vi "MultiChannelfFeedbackCooling (FPGA).vi"() -> ()   [LabVIEW 2016]
doc: "This VI will read single point values from 4 channels of a R Series board at a specified rate."
uses:
  <vilib>/rvi/Emulation/niFpgaGetClockAttributes.vi
  <vilib>/rvi/Emulation/niFpgaSctlEmulationGetInTimedLoop.vi
  <vilib>/rvi/Emulation/niFpgaEmulationReportErrorSimple.vi
  <vilib>/rvi/eio/common/nirviEmuTemplateMethod_errors.vi
  <vilib>/rvi/Memory/Memory_Emulation/nirvimemoryFastEmulation.vi
  <vilib>/rvi/Memory/Memory_Emulation/nirvimemoryEmulation.vi
  <vilib>/rvi/Emulation/niFpgaEmulationIsFPGAContextNoSignature.vi
  <vilib>/rvi/DataTransferAndStorage/Container/Common/niFpgaContainerGetUniqueNameForEmu.vi
  <vilib>/rvi/Emulation/niFpgaProcessEmulError.vi
  <vilib>/rvi/errors/nirviReportUnexpectedCaseInternalError (U32).vi
  <vilib>/rvi/Memory/Memory_Emulation/niFpgaMemoryEmulationCacheClearOnFirstRun.vi
  <vilib>/rvi/Memory/Memory_Emulation/nirvimemoryEmulationManagerCache_MakeExclusive.vi
  <vilib>/rvi/Memory/Memory_Emulation/niFpgaMemoryEmulationValidateCache.vi
  <vilib>/rvi/Memory/Memory_Emulation/nirvimemoryEmulationManagerCache_InsertValue.vi
  <vilib>/Utility/error.llb/Clear Errors.vi
  <vilib>/rvi/Memory/Memory_Emulation/nirvimemoryEmulationManagerCache_ReleaseExclusive.vi
  <vilib>/rvi/Memory/Memory_Emulation/nirvimemoryEmulationManagerCache_GetValue.vi
  <vilib>/rvi/Memory/Memory_Emulation/nirvimemoryEmulationManagerCache_SetValue.vi
  <vilib>/rvi/Emulation/niFpgaSctlEmulationResourceMgr.vi
  <vilib>/rvi/Emulation/niFpgaCriticalErrorInLSC.vi
  <vilib>/eio/EIONode/EIONode.xnode
  <vilib>/rvi/DataTransferAndStorage/Container/XNode/niFpgaContainer.xnode
  <vilib>/rvi/FXPMathLib/FxpInterpret/XNode/nifxpmath_Interpret.xnode
panel:
  in  "pg d0 1":fxp<+/-,24,12>
  in  "dg d0 1":fxp<+/-,24,12>
  in  "ig d0 1":fxp<+/-,24,6>
  in  "Upper lim d0 1":fxp<+/-,16,16>
  in  "Lower lim 2a":fxp<+/-,16,16>
  out "AI3":i16
  in  "lp coeff d0":i32[](array[numeric])=[1008310688, 32715568]
  in  "hp coeff d0":i32[](array[numeric])=[946630756, 1010186290]
  in  "Dc Pos d0":i16
  out "fb_d0":i16
  in  "Use_PID0_X":bool
  out "AI4":i16
  in  "Use_PID1_X":bool
  in  "Dc Pos d1":i16
  out "fb_d1":i16
  in  "Lower lim 3":fxp<+/-,16,16>
  in  "Upper lim d0 2":fxp<+/-,16,16>
  in  "pg d0 2":fxp<+/-,24,12>
  in  "hp coeff d1":i32[](array[numeric])=[946630756, 1010186290]
  in  "dg d0 2":fxp<+/-,24,12>
  in  "ig d0 2":fxp<+/-,24,6>
  in  "lp coeff d1":i32[](array[numeric])=[1008310688, 32715568]
  in  "ig 0":fxp<+/-,24,6>
  in  "pg 0":fxp<+/-,24,12>
  in  "ig 1":fxp<+/-,24,6>
  in  "pg 1":fxp<+/-,24,12>
  in  "pg_img":fxp<+/-,24,12>
  in  "dg_img":fxp<+/-,24,12>
  in  "ig_img":fxp<+/-,24,6>
  in  "setpt_img":i16
  out "AI_img":i16
  in  "lp coeff_img":i32[](array[numeric])=[1008310688, 32715568]
  in  "Upper lim_img":fxp<+/-,16,16>
  in  "Lower lim_img":fxp<+/-,16,16>
  in  "lp coeff d2":i32[](array[numeric])=[1008310688, 32715568]
  in  "hp coeff_img":i32[](array[numeric])=[946630756, 1010186290]
  out "tot_fb_img":i16
  out "fb_img":i16
  in  "output offset_img":i16
  in  "lp coeff 2":i32[](array[numeric])=[1008310688, 32715568]
  in  "data_buffer3":i16
  in  "Arb gain (ch2)":fxp<+/-,24,12>=0.5 caption="RMS"
  in  "lp coeff 0":i32[](array[numeric])=[1008310688, 32715568]
  in  "lp coeff 1":i32[](array[numeric])=[1008310688, 32715568]
  in  "hp coeff d2":i32[](array[numeric])=[946630756, 1010186290]
  in  "hp coeff 2":i32[](array[numeric])=[946630756, 1010186290]
  in  "hp coeff 1":i32[](array[numeric])=[946630756, 1010186290]
  in  "hp coeff 0":i32[](array[numeric])=[946630756, 1010186290]
  in  "Use_PID2_X 2":bool
  out "AI5":i16
  in  "Dc Pos d2":i16
  out "tot_fb_2":i16
  out "tot_fb_1":i16
  out "tot_fb_0":i16
  out "fb_d2":i16
  in  "output offset 2":i16
  in  "output offset 1":i16
  in  "output offset 0":i16
  in  "Lower lim 4":fxp<+/-,16,16>
  in  "Upper lim d0 3":fxp<+/-,16,16>
  in  "pg d0 3":fxp<+/-,24,12>
  in  "ig d03":fxp<+/-,24,6>
  in  "dg d0 3":fxp<+/-,24,12>
  out "fb_2":i16
  in  "ig 3":fxp<+/-,24,6>
  out "written_address":u32
  in  "ready_to_write":bool
  in  "Arb steps per cycle":u16
  in  "data_buffer2":i16
  in  "data_buffer_1":i16
  in  "write_address":u16
  in  "Arb gain (ch1)":fxp<+/-,24,12>=0.5 caption="RMS"
  in  "Arb gain (ch0)":fxp<+/-,24,12>=0.5 caption="RMS"
  out "fb_1":i16
  out "fb_0":i16
  in  "Dc Pos 1":i16
  in  "Dc Pos 0":i16
  in  "Lower lim 2":fxp<+/-,16,16>
  in  "Upper lim 2":fxp<+/-,16,16>
  in  "dg 2":fxp<+/-,24,12>
  in  "pg 2":fxp<+/-,24,12>
  out "AI2":i16
  in  "Dc Pos 2":i16
  out "AI1":i16
  in  "dg 1":fxp<+/-,24,12>
  in  "Upper lim 1":fxp<+/-,16,16>
  in  "Lower lim 1":fxp<+/-,16,16>
  out "AI0":i16
  in  "dg 0":fxp<+/-,24,12>
  in  "Upper lim 0":fxp<+/-,16,16>
  in  "Lower lim 0":fxp<+/-,16,16>
  in  "Count(uSec)":u32
  out "FPGA Error Out":errorcluster
  in  "Stop":bool
  # "test"
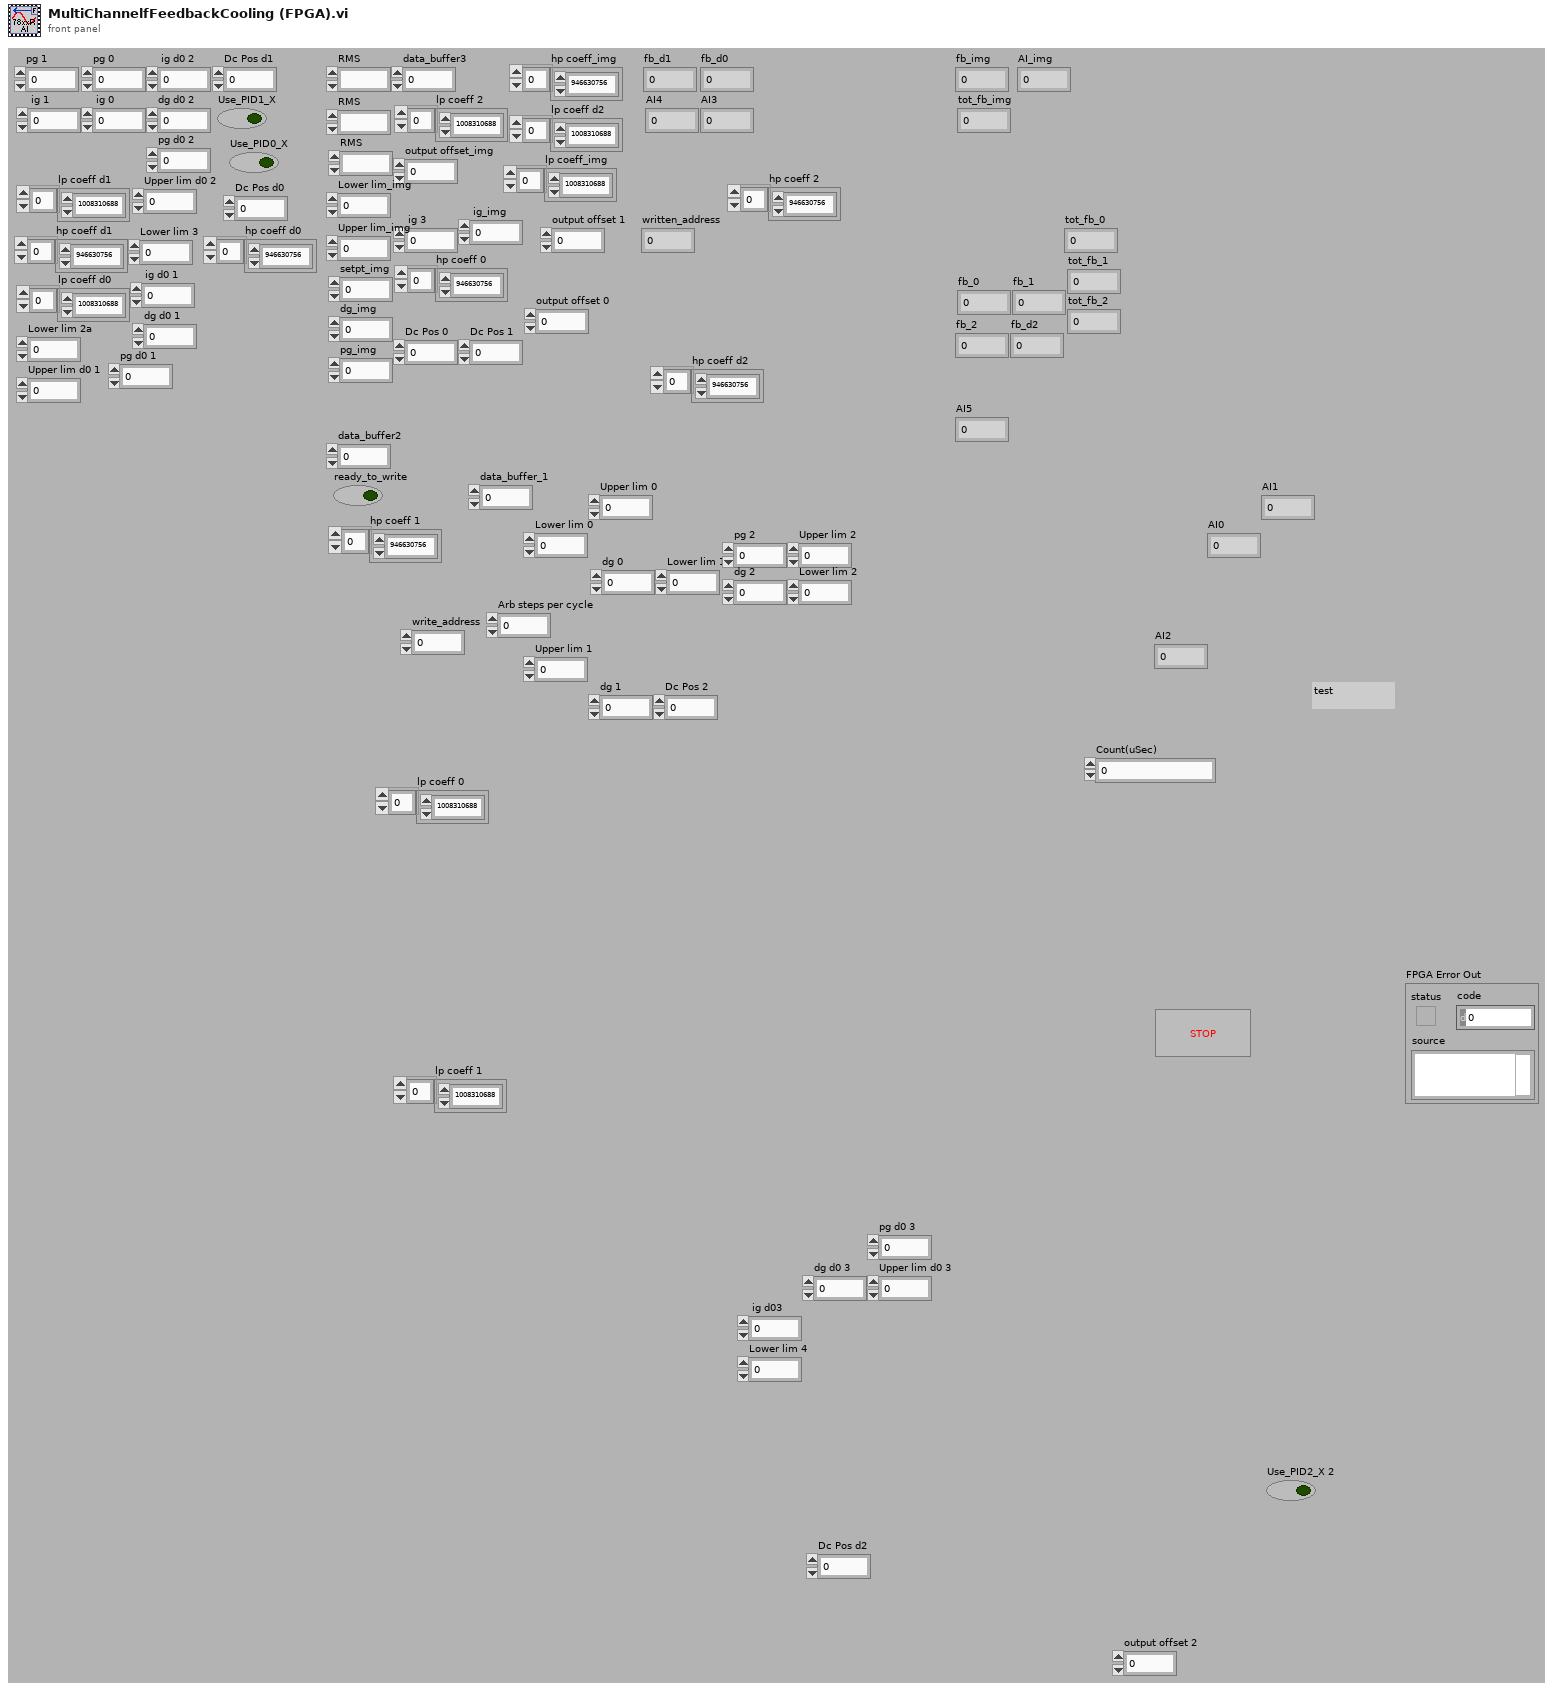
[diagram p1: front panel]
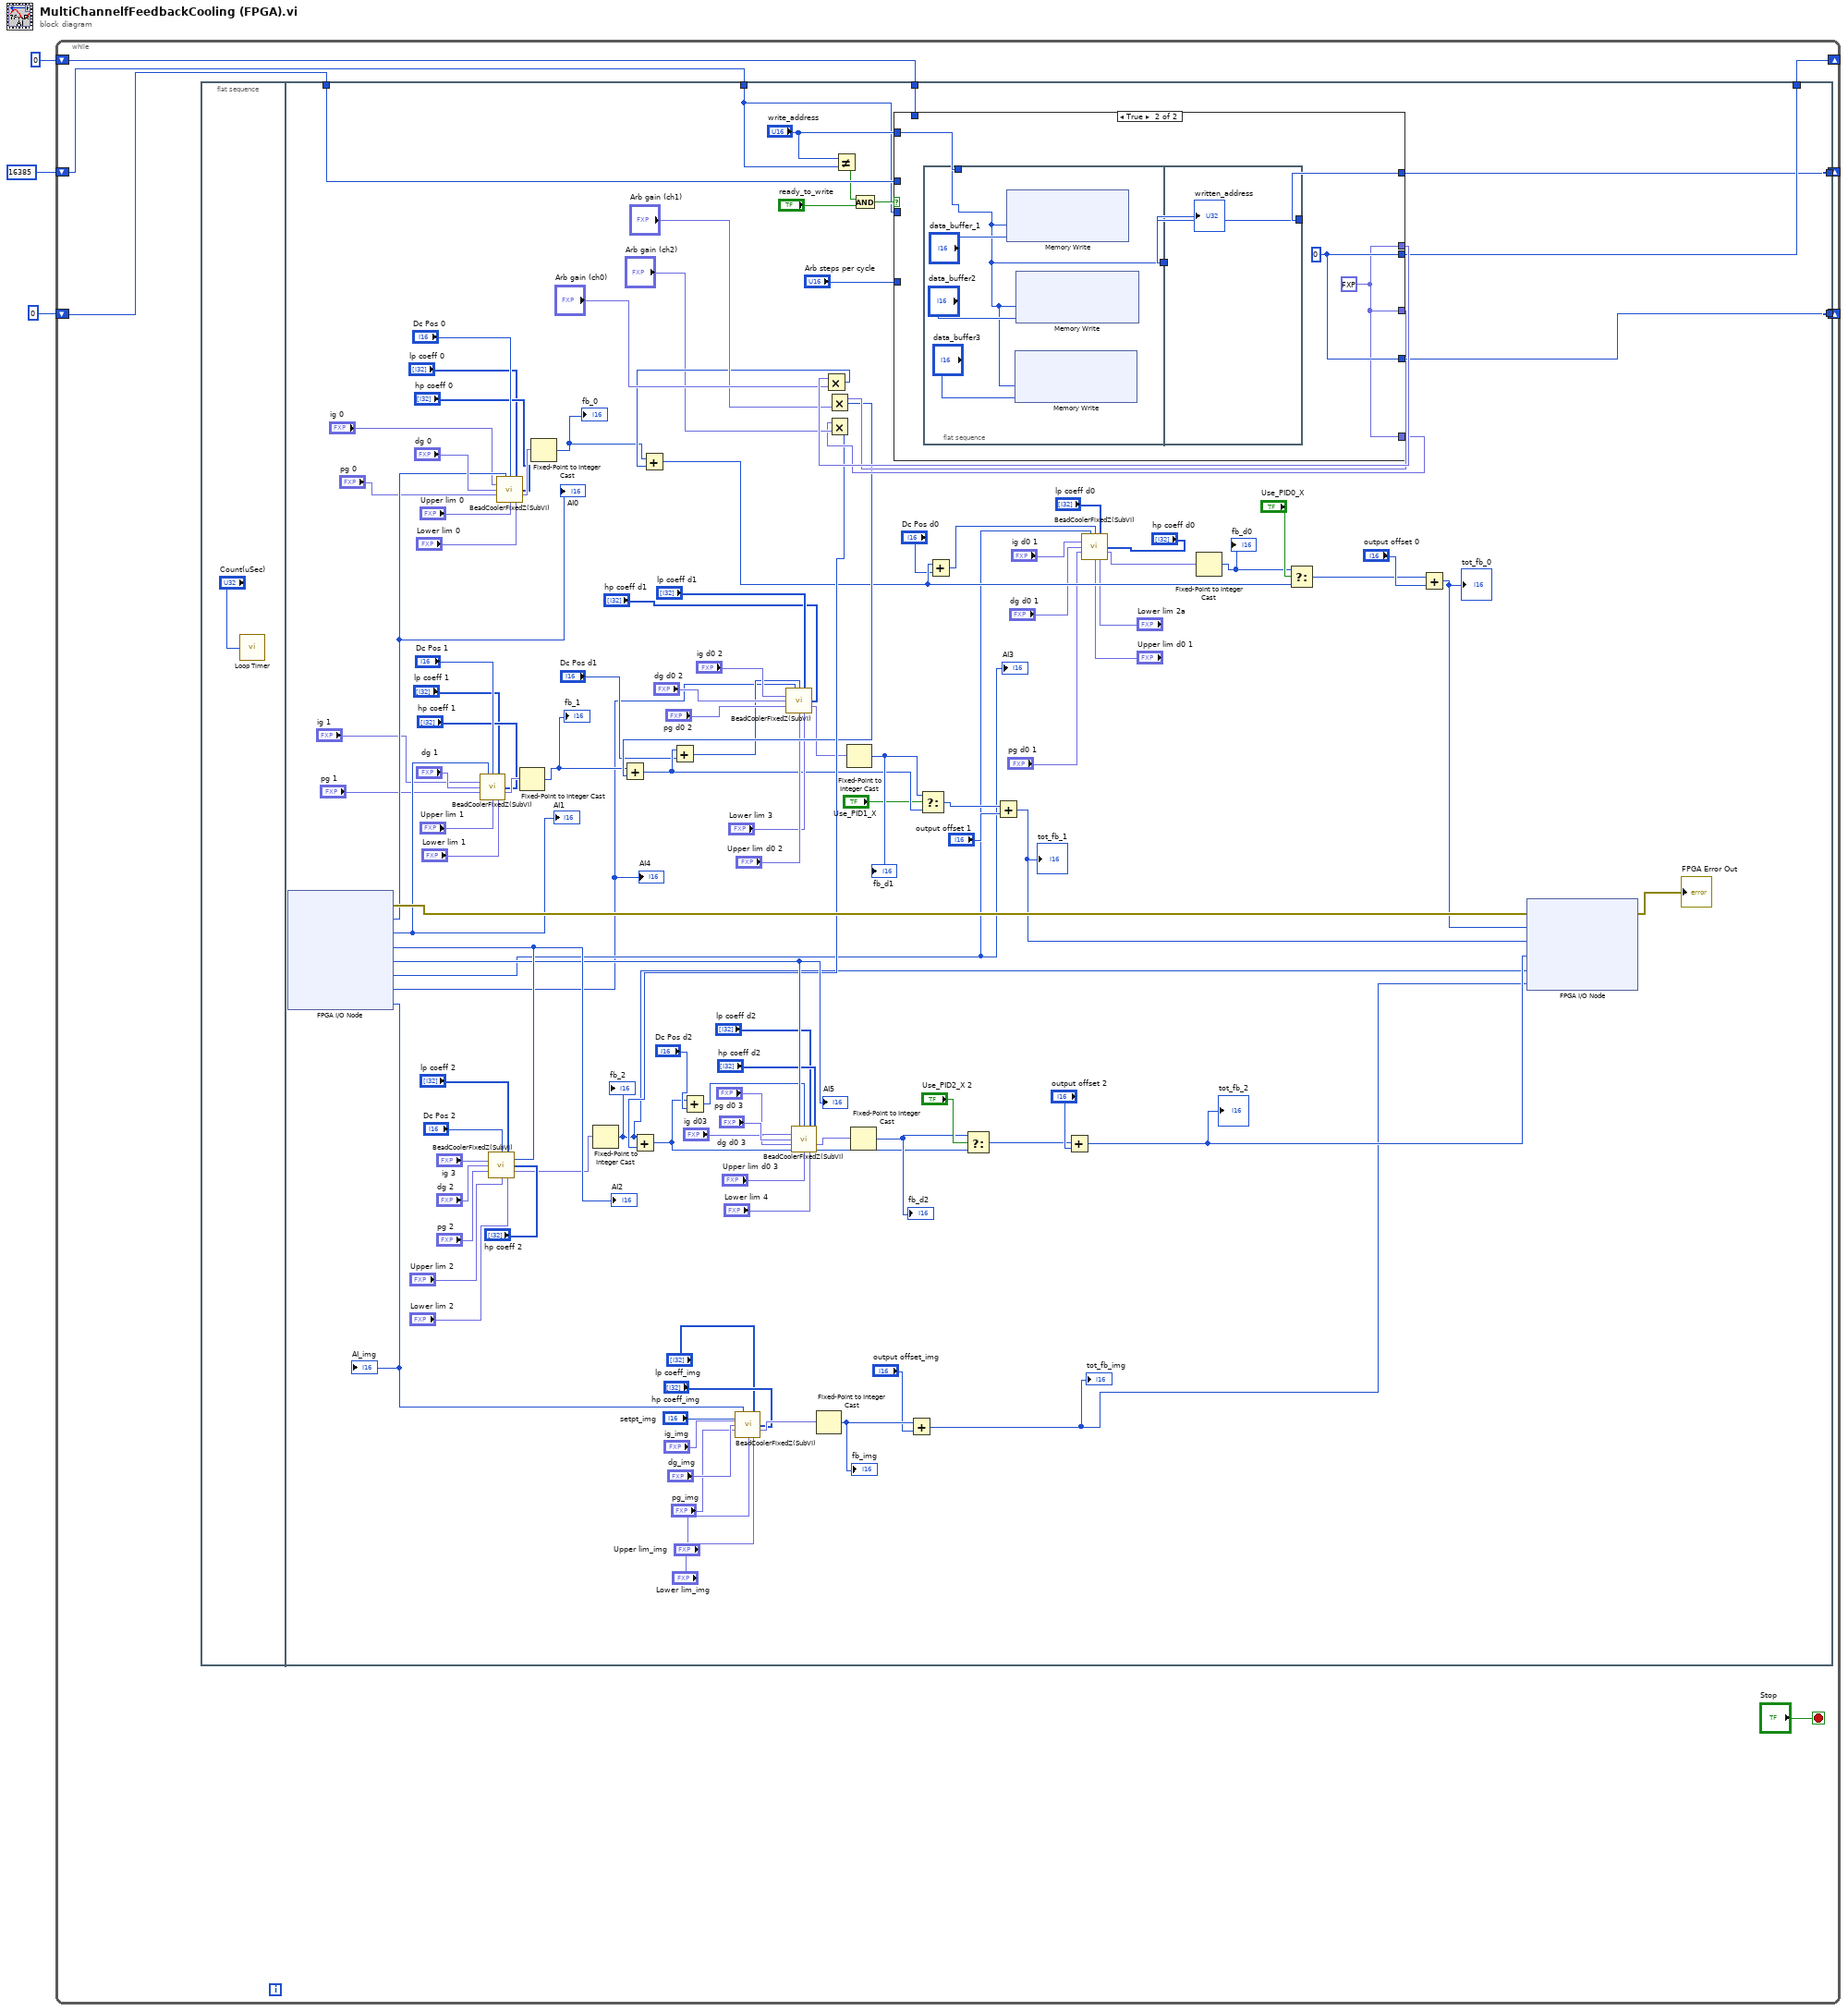
[diagram p0: block diagram]
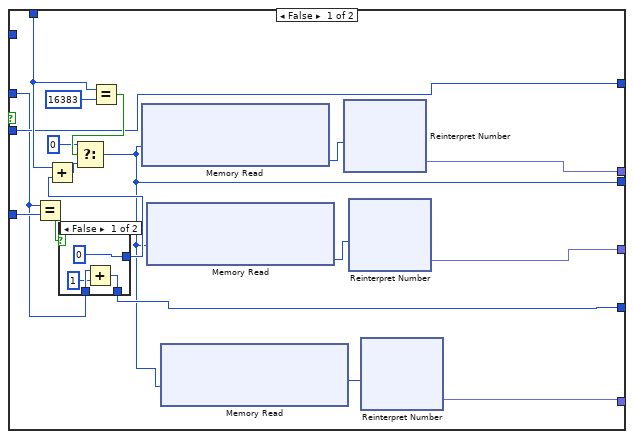
[diagram p2: hidden frame]
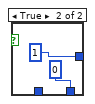
[diagram p3: hidden frame]
diagram:
  n1 = while {
    shift-right: [w9] -> _
    shift-left: u16 0 ("t") -> [w8]
    shift-right: [w7] -> _
    shift-left: u16 0 ("t") -> [w4]
    shift-right: [w6] -> _
    shift-left: u32 16385 ("write_address") -> [w5]
    stop <- "Stop" stop-if-true
    n2 = flat-sequence {
      tunnel: [w113] -> w9
      tunnel: w8 -> [w112]
      tunnel: [w110] -> w7
      tunnel: w4 -> [w109]
      tunnel: [w108] -> w6
      tunnel: w5 -> [w100]
      frame #0 {
        n3 = call "Loop Timer"("Count(uSec)"="Count(uSec)") -> ()  [unwired: 1 out]
      }
      frame #1 {
        n4 = xnode "FPGA I/O Node"() -> ("error out"=w130:errorcluster, "Connector0/AI0"=w99:i16, "Connector0/AI1"=w98:i16, "Connector0/AI2"=w95:i16, "Connector0/AI5"=w83:i16, "Connector0/AI3"=w18:i16, "Connector0/AI4"=w12:i16, "Connector0/AI6"=w49:i16)  [unwired: 8 in, 7 out]
        "AI0" <- w99
        "AI1" <- w98
        "AI2" <- w95
        "AI5" <- w83
        "AI_img" <- w49
        "AI4" <- w12
        "AI3" <- w18
        n5 = call "BeadCoolerFixedZ(SubVI).vi"("AI0"=w98, "Dc Pos"="Dc Pos 1", "lp coeff"="lp coeff 1", "ig"="ig 1", "dg"="dg 1", "hp coeff"="hp coeff 1", "pg"="pg 1", "Upper lim"="Upper lim 1", "Lower lim"="Lower lim 1") -> ("Output"=w97:fxp<+/-,16,16>)  [unwired: 6 in]
        n6 = call "BeadCoolerFixedZ(SubVI).vi"("AI0"=w95, "Dc Pos"="Dc Pos 2", "lp coeff"="lp coeff 2", "ig"="ig 3", "dg"="dg 2", "hp coeff"="hp coeff 2", "pg"="pg 2", "Upper lim"="Upper lim 2", "Lower lim"="Lower lim 2") -> ("Output"=w73:fxp<+/-,16,16>)  [unwired: 6 in]
        n7 = call "BeadCoolerFixedZ(SubVI).vi"("AI0"=w99, "Dc Pos"="Dc Pos 0", "lp coeff"="lp coeff 0", "ig"="ig 0", "dg"="dg 0", "hp coeff"="hp coeff 0", "pg"="pg 0", "Upper lim"="Upper lim 0", "Lower lim"="Lower lim 0") -> ("Output"=w101:fxp<+/-,16,16>)  [unwired: 6 in]
        n8 = Fixed-Point to Integer Cast(1:w97) -> (0:w30:i16)
        "fb_1" <- w30
        n9 = Fixed-Point to Integer Cast(1:w101) -> (0:w68:i16)
        "fb_0" <- w68
        n10 = Fixed-Point to Integer Cast(1:w73) -> (0:w36:i16)
        "fb_2" <- w36
        n11 = call "BeadCoolerFixedZ(SubVI).vi"("AI0"=w49, "Dc Pos"="setpt_img", "lp coeff"="lp coeff_img", "ig"="ig_img", "dg"="dg_img", "hp coeff"="hp coeff_img", "pg"="pg_img", "Upper lim"="Upper lim_img", "Lower lim"="Lower lim_img") -> ("Output"=w62:fxp<+/-,16,16>)  [unwired: 6 in]
        n12 = Fixed-Point to Integer Cast(1:w62) -> (0:w61:i16)
        "fb_img" <- w61
        n13 = Not Equal?(x="write_address", y=w100) -> (x != y?=w105:bool)
        n14 = And(x=w105, y="ready_to_write") -> (x .and. y?=w106:bool)
        n15 = case shown="True" w106 {
          tunnel: [w147 w155] -> w115
          tunnel: [w132 w159] -> w113
          tunnel: w112 -> [w140 _]
          tunnel: [w141 w155] -> w103
          tunnel: "Arb steps per cycle" -> [w139 _]
          tunnel: [w134 w159] -> w110
          tunnel: w109 -> [w135 _]
          tunnel: [w138 w157] -> w108
          tunnel: w100 -> [w138 _]
          tunnel: "write_address" -> [_ w156]
          tunnel: [w131 w155] -> w66
          frame False {
            n16 = Equal?(x=w135, y=w139) -> (x = y?=w137:bool)
            n17 = case shown="False" w137 {
              tunnel: [u16 0 ("y") u16 1 ("y")] -> w136
              tunnel: w135 -> [w151 _]
              tunnel: [w149 u16 0] -> w134
              frame False {
                n18 = Add(x=w151, y=u16 1) -> (x+y=w149:u16)
              }
              frame True {
              }
            }
            n19 = Add(x=w140, y=w136) -> (x+y=w143:u16)
            n20 = Equal?(x=w140, y=u16 16383) -> (x = y?=w145:bool)
            n21 = Select(t=u16 0, s=w145, f=w143) -> (s? t:f=w132:u16)
            n22 = xnode ("Memory Read")("Address"=w132) -> ("Data"=w148:i16)  [unwired: 1 in, 1 out]
            n23 = xnode ("Memory Read")("Address"=w132) -> ("Data"=w142:i16)  [unwired: 1 in, 1 out]
            n24 = xnode ("Memory Read")("Address"=w132) -> ("Data"=w133:i16)  [unwired: 1 in, 1 out]
            n25 = xnode "Reinterpret Number"("x"=w148) -> ("y"=w147:fxp<+/-,16,16>)
            n26 = xnode "Reinterpret Number"("x"=w142) -> ("y"=w141:fxp<+/-,16,16>)
            n27 = xnode "Reinterpret Number"("x"=w133) -> ("y"=w131:fxp<+/-,16,16>)
          }
          frame True {
            w159 = u16 0
            w155 = fxp<+/-,16,16> 0.0 ("y")
            n28 = flat-sequence {
              tunnel: [w161] -> w158
              tunnel: w156 -> [w161]
              tunnel: w158 -> [w164]
              tunnel: [w164] -> w157
              frame #0 {
                n29 = xnode ("Memory Write")("Address"=w161, "Data"="data_buffer_1") -> ()  [unwired: 1 in, 1 out]
                n30 = xnode ("Memory Write")("Address"=w161, "Data"="data_buffer3") -> ()  [unwired: 1 in, 1 out]
                n31 = xnode ("Memory Write")("Address"=w161, "Data"="data_buffer2") -> ()  [unwired: 1 in, 1 out]
              }
              frame #1 {
                "written_address" <- w164
              }
            }
          }
        }
        n32 = Multiply(x=w115, y="Arb gain (ch0)") -> (x*y=w87:i16)
        n33 = Add(x=w68, y=w87) -> (x+y=w22:i16)
        n34 = Multiply(x=w103, y="Arb gain (ch1)") -> (x*y=w64:i16)
        n35 = Add(x=w30, y=w64) -> (x+y=w33:i16)
        n36 = Add(x=w33, y="Dc Pos d1") -> (x+y=w31:i16)
        n37 = call "BeadCoolerFixedZ(SubVI).vi"("AI0"=w12, "Dc Pos"=w31, "lp coeff"="lp coeff d1", "ig"="ig d0 2", "dg"="dg d0 2", "hp coeff"="hp coeff d1", "pg"="pg d0 2", "Upper lim"="Upper lim d0 2", "Lower lim"="Lower lim 3") -> ("Output"=w37:fxp<+/-,16,16>)  [unwired: 6 in]
        n38 = Multiply(x=w66, y="Arb gain (ch2)") -> (x*y=w65:i16)
        n39 = Add(x=w36, y=w65) -> (x+y=w72:i16)
        n40 = Add(x=w72, y="Dc Pos d2") -> (x+y=w69:i16)
        n41 = call "BeadCoolerFixedZ(SubVI).vi"("AI0"=w83, "Dc Pos"=w69, "lp coeff"="lp coeff d2", "ig"="ig d03", "dg"="dg d0 3", "hp coeff"="hp coeff d2", "pg"="pg d0 3", "Upper lim"="Upper lim d0 3", "Lower lim"="Lower lim 4") -> ("Output"=w89:fxp<+/-,16,16>)  [unwired: 6 in]
        n42 = Fixed-Point to Integer Cast(1:w37) -> (0:w34:i16)
        "fb_d1" <- w34
        n43 = Fixed-Point to Integer Cast(1:w89) -> (0:w80:i16)
        "fb_d2" <- w80
        n44 = Add(x=w61, y="output offset_img") -> (x+y=w60:i16)
        "tot_fb_img" <- w60
        n45 = Select(t=w34, s="Use_PID1_X", f=w33) -> (s? t:f=w35:i16)
        n46 = Add(x=w22, y="Dc Pos d0") -> (x+y=w23:i16)
        n47 = Select(t=w80, s="Use_PID2_X 2", f=w72) -> (s? t:f=w79:i16)
        n48 = Add(x=w35, y="output offset 1") -> (x+y=w81:i16)
        "tot_fb_1" <- w81
        n49 = Add(x=w79, y="output offset 2") -> (x+y=w78:i16)
        "tot_fb_2" <- w78
        n50 = call "BeadCoolerFixedZ(SubVI).vi"("AI0"=w18, "Dc Pos"=w23, "lp coeff"="lp coeff d0", "ig"="ig d0 1", "dg"="dg d0 1", "hp coeff"="hp coeff d0", "pg"="pg d0 1", "Upper lim"="Upper lim d0 1", "Lower lim"="Lower lim 2a") -> ("Output"=w24:fxp<+/-,16,16>)  [unwired: 6 in]
        n51 = Fixed-Point to Integer Cast(1:w24) -> (0:w25:i16)
        "fb_d0" <- w25
        n52 = Select(t=w25, s="Use_PID0_X", f=w22) -> (s? t:f=w26:i16)
        n53 = Add(x=w26, y="output offset 0") -> (x+y=w28:i16)
        "tot_fb_0" <- w28
        n54 = xnode "FPGA I/O Node"("error in"=w130, "Connector0/AO0"=w28, "Connector0/AO1"=w81, "Connector0/AO2"=w78, "Connector0/AO3"=w36, "Connector0/AO4"=w60) -> ("error out"=→"FPGA Error Out":errorcluster)  [unwired: 5 in, 5 out]
      }
    }
  }
